vi "read_and_write.vi"() -> ()   [LabVIEW 2012]
panel:
  out "x = y?":bool
  out "Read_output":u8[](array[numeric])
  out "buffer":u8[](array[numeric])
  out "return type 3":i32
  out "length out 1":i32
  out "string Out":string
  out "Length to Write":u32
  out "return type 2":i32
  out "return type":i32
  out "text":string
  in  "file (use dialog)":path
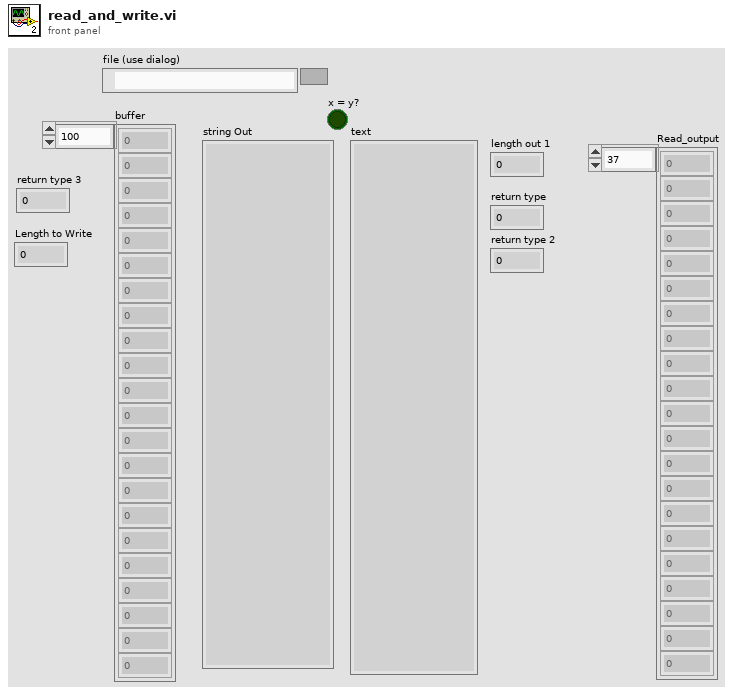
[diagram p1: front panel]
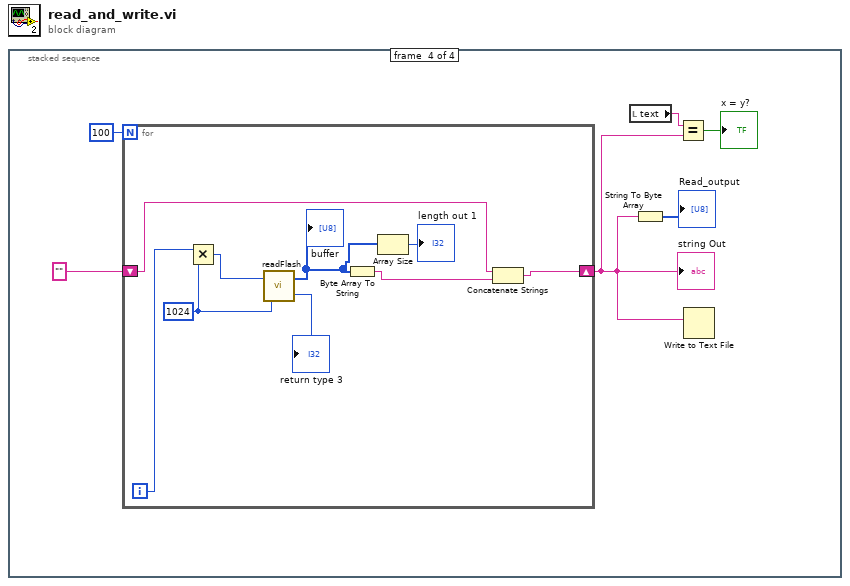
[diagram p0: block diagram]
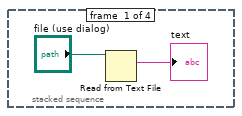
[diagram p2: hidden frame]
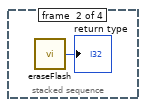
[diagram p3: hidden frame]
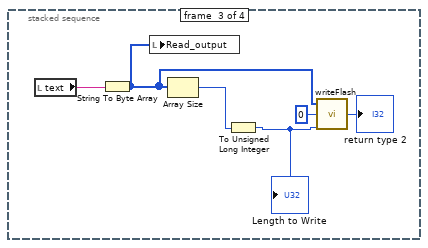
[diagram p4: hidden frame]
diagram:
  n1 = stacked-sequence {
    frame #0 {
      n2 = Read from Text File(file (use dialog)="file (use dialog)") -> (text=→"text":string)  [unwired: 3 in, 3 out]
    }
    frame #1 {
      n3 = call "eraseFlash.vi"() -> ("return type"=→"return type":i32)
    }
    frame #2 {
      n4 = local read "text"() -> (w5:string)
      n5 = String To Byte Array(string=w5) -> (unsigned byte array=w4:u8[])
      n6 = local write "Read_output"(w4) -> ()
      n7 = Array Size(array=w4) -> (size(s)=w8:i32)
      n8 = To Unsigned Long Integer(number=w8) -> (unsigned 32bit integer=w7:u32)
      "Length to Write" <- w7
      n9 = call "writeFlash.vi"("bytesToWrite"=w7, "offset"=u32 0, "buffer"=w4) -> ("return type"=→"return type 2":i32)
    }
    frame #3 {
      n10 = for {
        N: 100 -> [_]
        shift-right: [w17] -> w12
        shift-left: "" -> [w19]
        i -> [w20]
        w21 = u16 1024 ("bytesToRead")
        n11 = Multiply(x=w20, y=w21) -> (x*y=w16:i32)
        n12 = call "readFlash.vi"("bytesToRead"=w21, "offset"=w16) -> ("return type"=→"return type 3":i32, "buffer"=w23:u8[])
        "buffer" <- w23
        n13 = Byte Array To String(unsigned byte array=w23) -> (string=w18:string)
        n14 = Array Size(array=w23) -> (size(s)=→"length out 1":i32)
        n15 = Concatenate Strings(w19, w18) -> (w17:string)
      }
      "string Out" <- w12
      n16 = local read "text"() -> (w11:string)
      n17 = String To Byte Array(string=w12) -> (unsigned byte array=→"Read_output":u8[])
      n18 = Equal?(x=w11, y=w12) -> (x = y?=→"x = y?":bool)
      n19 = Write to Text File(text=w12) -> ()  [unwired: 3 in, 3 out]
    }
  }
